vi "loadDataNodeBegin.vi"(8 "error in (no error)":errorcluster, 10 "XML Refnum in":refnum<file>, 11 "DMA_Read in":refnum<class "DMA_Read.lvclass">) -> (0 "error out":errorcluster, 2 "XML Refnum out":refnum<file>, 3 "DMA_Read out":refnum<class "DMA_Read.lvclass">)   [LabVIEW 2013, in "DMA_Read.lvclass"]
doc: "Part of the file loading process. Occurs at the beginning of a node being loaded. Loads the common xceDataNode data name and description."
uses:
  DMA_Read.lvclass
  DMA_Read.lvclass/DMA_Read.ctl
  XML Parser/XML Parser.lvclass
  xCE/xceNode/xceNode.lvclass
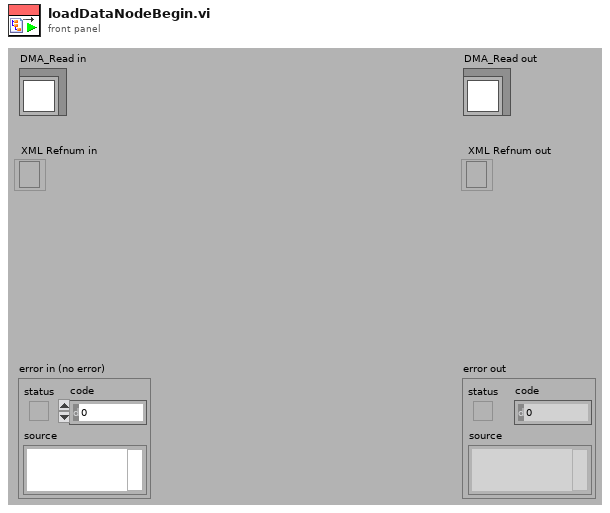
[diagram p1: front panel]
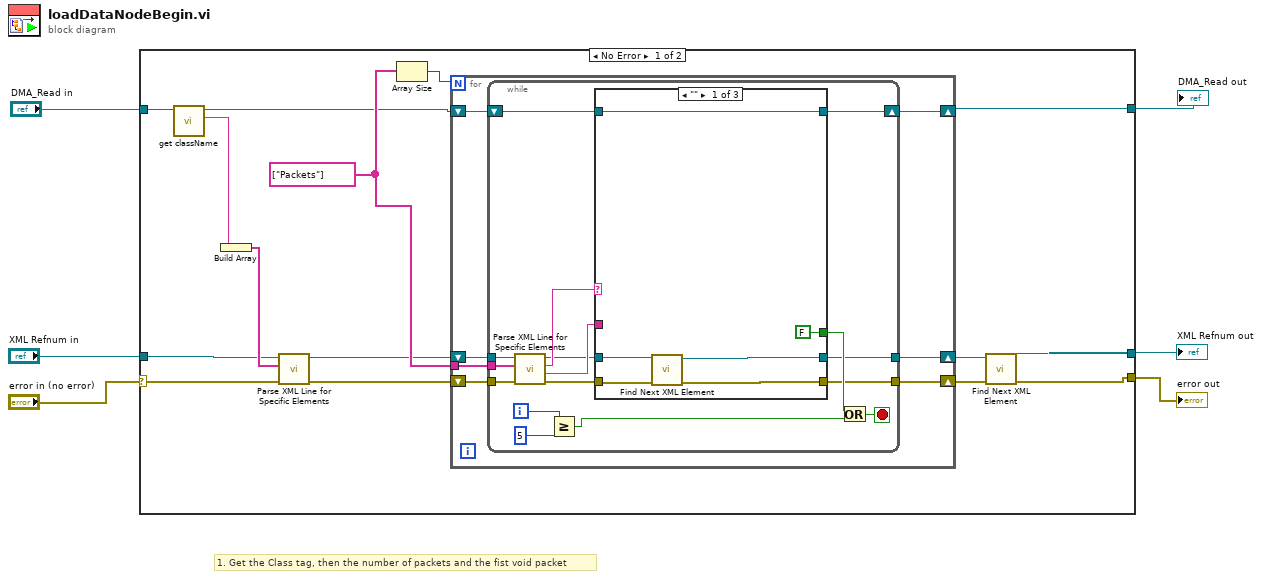
[diagram p0: block diagram]
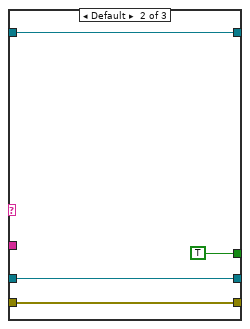
[diagram p2: hidden frame]
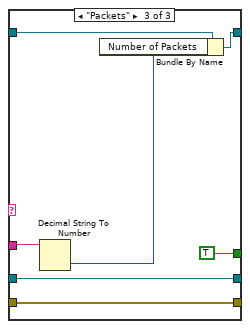
[diagram p3: hidden frame]
diagram:
  # "1. Get the Class tag, then the number of packets and the fist void packet"
  n1 = case shown="No Error" "error in (no error)" {
    selector: "error in (no error)" -> [w13 w64]
    tunnel: [w8 w64] -> w2
    tunnel: [w19 w63] -> w1
    tunnel: [w7 w62] -> w3
    tunnel: "DMA_Read in" -> [w17 w63]
    tunnel: "XML Refnum in" -> [w14 w62]
    frame No Error {
      w20 = string[] ["Packets"] ("Token List")
      n2 = call "get className.vi"("xceNode in"=w17) -> ("Class name"=w15:string, "xceNode out"=w16:refnum<class "DMA_Read.lvclass">)  [unwired: 8 in, 1 out]
      n3 = Build Array(w15) -> (w18:string[])
      n4 = call "Parse XML Line for Specific Elements.vi"("error in (no error)"=w13, "Elements"=w18, "XML Refnum in"=w14) -> ("error out"=w11:errorcluster, "XML Refnum out"=w12:refnum<file>)  [unwired: 4 in, 3 out]
      n5 = Array Size(array=w20) -> (size(s)=w21:i32)
      n6 = for {
        N: w21 -> [_]
        tunnel: w20 -> [w28]
        shift-right: [w23] -> w19
        shift-left: w16 -> [w25]
        shift-right: [w24] -> w10
        shift-left: w12 -> [w27]
        shift-right: [w22] -> w9
        shift-left: w11 -> [w26]
        n7 = while {
          tunnel: w28 -> [w44]
          tunnel: w27 -> [w43]
          tunnel: w26 -> [w42]
          shift-right: [w37] -> w23
          shift-left: w25 -> [w39]
          tunnel: [w29] -> w24
          tunnel: [w30] -> w22
          i -> [w41]
          stop <- w34 stop-if-true
          n8 = call "Parse XML Line for Specific Elements.vi"("error in (no error)"=w42, "Elements"=w44, "XML Refnum in"=w43) -> ("error out"=w31:errorcluster, "Value"=w33:string, "Element Name"=w38:string, "XML Refnum out"=w32:refnum<file>)  [unwired: 4 in, 1 out]
          n9 = Greater Or Equal?(x=w41, y=5) -> (x >= y?=w35:bool)
          n10 = case shown="\"\"" w38 {
            tunnel: w39 -> [w50 w54 w61]
            tunnel: [w50 w54 w60] -> w37
            tunnel: [FALSE TRUE TRUE] -> w36
            tunnel: w33 -> [_ _ w56]
            tunnel: w32 -> [w48 w52 w58]
            tunnel: w31 -> [w47 w51 w57]
            tunnel: [w45 w51 w57] -> w30
            tunnel: [w46 w52 w58] -> w29
            frame "" {
              n11 = call "Find Next XML Element.vi"("error in (no error)"=w47, "XML Fine In"=w48) -> ("error out"=w45:errorcluster, "XML Fine Out"=w46:refnum<file>)  [unwired: 7 in, 1 out]
            }
            frame Default {
            }
            frame "Packets" {
              n12 = Decimal String To Number(string=w56) -> (number=w55:i32)  [unwired: 2 in, 1 out]
              n13 = Bundle By Name(cluster=w61, "Number of Packets"=w55) -> (w60:refnum<class "DMA_Read.lvclass">)
            }
          }
          n14 = Or(x=w36, y=w35) -> (x .or. y?=w34:bool)
        }
      }
      n15 = call "Find Next XML Element.vi"("error in (no error)"=w9, "XML Fine In"=w10) -> ("error out"=w8:errorcluster, "XML Fine Out"=w7:refnum<file>)  [unwired: 7 in, 1 out]
    }
    frame Error {
    }
  }
  "error out" <- w2
  "DMA_Read out" <- w1
  "XML Refnum out" <- w3
